vi "Close.vi"(8 "error in (no error)":errorcluster, 11 "Hardware in":refnum<class "Hardware.lvclass">) -> (0 "error out":errorcluster, 3 "Hardware out":refnum<class "Hardware.lvclass">)   [LabVIEW 2016, in "Hardware.lvclass"]
uses:
  Hardware.lvclass
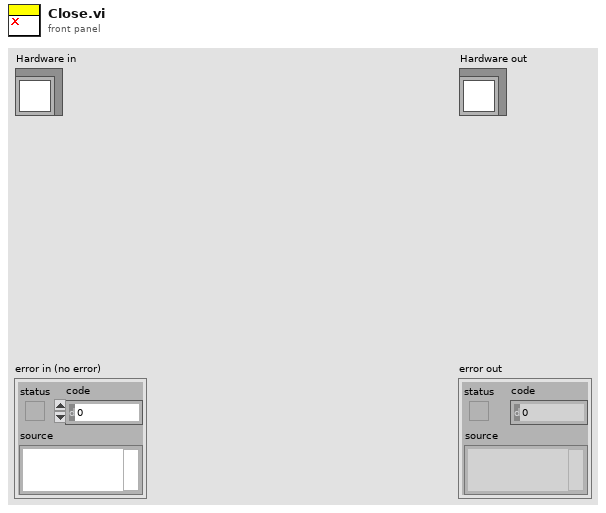
[diagram p1: front panel]
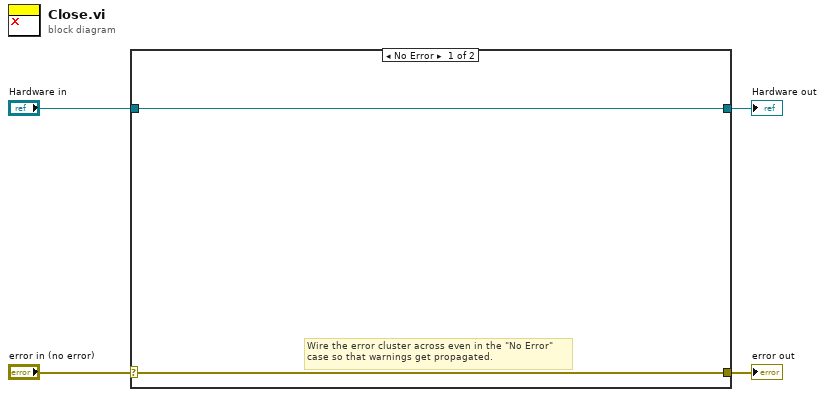
[diagram p0: block diagram]
diagram:
  n1 = case shown="No Error" "error in (no error)" {
    selector: "error in (no error)" -> [w5 w8]
    tunnel: [w5 w8] -> w3
    tunnel: [w6 w7] -> w1
    tunnel: "Hardware in" -> [w6 w7]
    frame No Error {
      # "Wire the error cluster across even in the \"No Error\"\ncase so that warnings get propagated."
    }
    frame Error {
    }
  }
  "error out" <- w3
  "Hardware out" <- w1
